vi "StabilizeAll.vi"() -> ()   [LabVIEW 2017]
panel:
  in  "Frame to Use for Template":i32=5000
  out "Horizontal Progress Bar":u8(slide) scale=0.0..49.0
  out "Stabilzing":dbl
  out "Total Video Segments to Stabilize":dbl
  # "This VI stabilizes all AVI videos in the selected folder. The user is prompted to select the folder after which they are asked to choose the region to be stabilized for each video. The program will then run automously to stabilize all the videos."
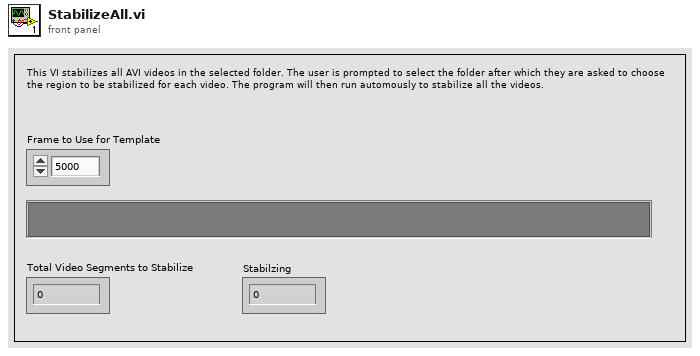
[diagram p1: front panel]
types:
  T1 = typedef "IMAQ AVI2 Refnum.ctl" = refnum<k20>
  T2 = typedef "IMAQ Image.ctl" = refnum<image>
  T3 = typedef "IMAQ Rectangle" = cluster{"Left":i32, "Top":i32, "Right":i32, "Bottom":i32, "Rotation":dbl}
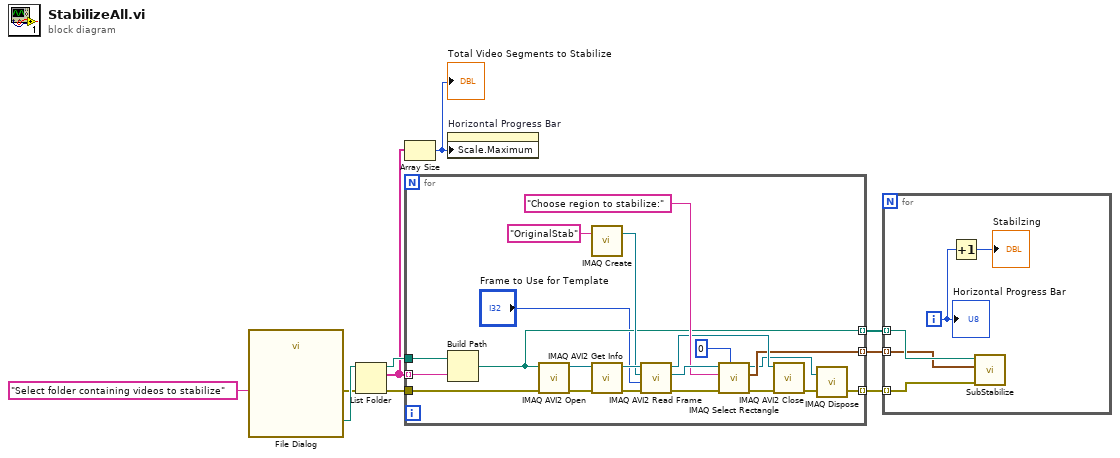
[diagram p0: block diagram]
diagram:
  n1 = call "File Dialog"("prompt"="Select folder containing videos to stabilize") -> ("selected path"=w9:path, "error out"=w8:errorcluster)  [unwired: 11 in, 2 out]
  n2 = List Folder(path=w9, error in=w8) -> (path out=w7:path, filenames=w2:string[], error out=w6:errorcluster)  [unwired: 2 in, 1 out]
  n3 = Array Size(array=w2) -> (size(s)=w1:i32)
  "Total Video Segments to Stabilize" <- w1
  n4 = for {
    tunnel: w7 -> [w31]
    tunnel: w2 -> [w30] mode=indexing
    tunnel: w6 -> [w19]
    tunnel: [w16] -> w5 mode=indexing
    tunnel: [w13] -> w4 mode=indexing
    tunnel: [w15] -> w3 mode=indexing
    n5 = Build Path(base path=w31, name or relative path=w30) -> (appended path=w15:path)
    n6 = call "IMAQ AVI2 Open"("error in (no error)"=w19, "AVI File Path"=w15) -> ("error out"=w28:errorcluster, "AVI Refnum"=w29:T1)  [unwired: 8 in]
    n7 = call "IMAQ Create"("Image Name"="OriginalStab") -> ("New Image"=w25:T2)  [unwired: 4 in, 1 out]
    n8 = call "IMAQ AVI2 Get Info"("error in (no error)"=w28, "AVI Refnum"=w29) -> ("error out"=w24:errorcluster, "AVI Refnum (duplicate)"=w27:T1)  [unwired: 5 in, 3 out]
    n9 = call "IMAQ AVI2 Read Frame"("error in (no error)"=w24, "Frame Number"="Frame to Use for Template", "Image"=w25, "AVI Refnum"=w27) -> ("error out"=w20:errorcluster, "Image Out"=w23:T2, "AVI Refnum (duplicate)"=w17:T1)  [unwired: 5 in]
    n10 = call "IMAQ Select Rectangle"("Window Number (0...15)"=0, "error in (no error)"=w20, "Prompt"="Choose region to stabilize:", "Image In"=w23) -> ("error out"=w18:errorcluster, "Rectangle"=w16:T3, "Image Out (duplicate)"=w12:T2)  [unwired: 4 in, 1 out]
    n11 = call "IMAQ AVI2 Close"("error in (no error)"=w18, "AVI Refnum"=w17) -> ("error out"=w14:errorcluster)  [unwired: 9 in]
    n12 = call "IMAQ Dispose"("Image"=w12, "error in (no error)"=w14) -> ("error out"=w13:errorcluster)  [unwired: 4 in]
  }
  n13 = property on="Horizontal Progress Bar" class="Slide (strict)"("Scale.Maximum"=w1) -> ()  [unwired: 2 in, 2 out]
  n14 = for {
    tunnel: w5 -> [w35] mode=indexing
    tunnel: w4 -> [w34] mode=indexing
    tunnel: w3 -> [w36] mode=indexing
    i -> [w33]
    n15 = Increment(x=w33) -> (x+1=→"Stabilzing":i32)
    n16 = call "SubStabilize.vi"("error in (no error)"=w34, "Rectangle"=w35, "path"=w36) -> ()  [unwired: 8 in, 1 out]
    "Horizontal Progress Bar" <- w33
  }
